vi "AddTargets.vi"(8 "error in (no error)":errorcluster, 9 "Difficulty":u8, 10 "Num Targets":i32, 11 "Level in":refnum<class "Level.lvclass">) -> (0 "error out":errorcluster, 3 "Level out":refnum<class "Level.lvclass">)   [LabVIEW 2015, in "Level.lvclass"]
uses:
  Level.lvclass
  Level.lvclass/Level.ctl
  Segment.ctl
  Point.ctl
  3D Point.ctl
  3D Object/3D Object.lvclass
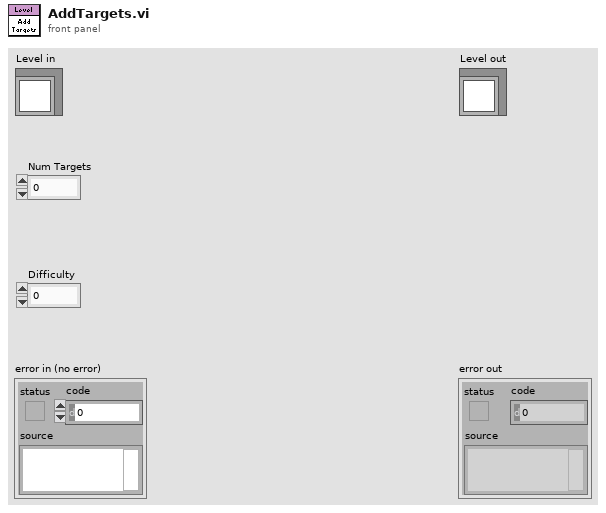
[diagram p1: front panel]
types:
  T1 = typedef "Level.lvclass/Segment.ctl" = cluster{"Point 1":T2, "Point 2":T2}
  T2 = typedef "Level.lvclass/Point.ctl" = cluster{"Z":dbl, "X":dbl}
  T3 = typedef "3D Point.ctl" = cluster{"X":sgl, "Y":sgl, "Z":sgl}
  T4 = cluster{"Collision":T1, "Position":T3, "Radius":dbl}
  T5 = enum16{"As a Decal", "With Modulation", "With Blending", "As a replacement"}
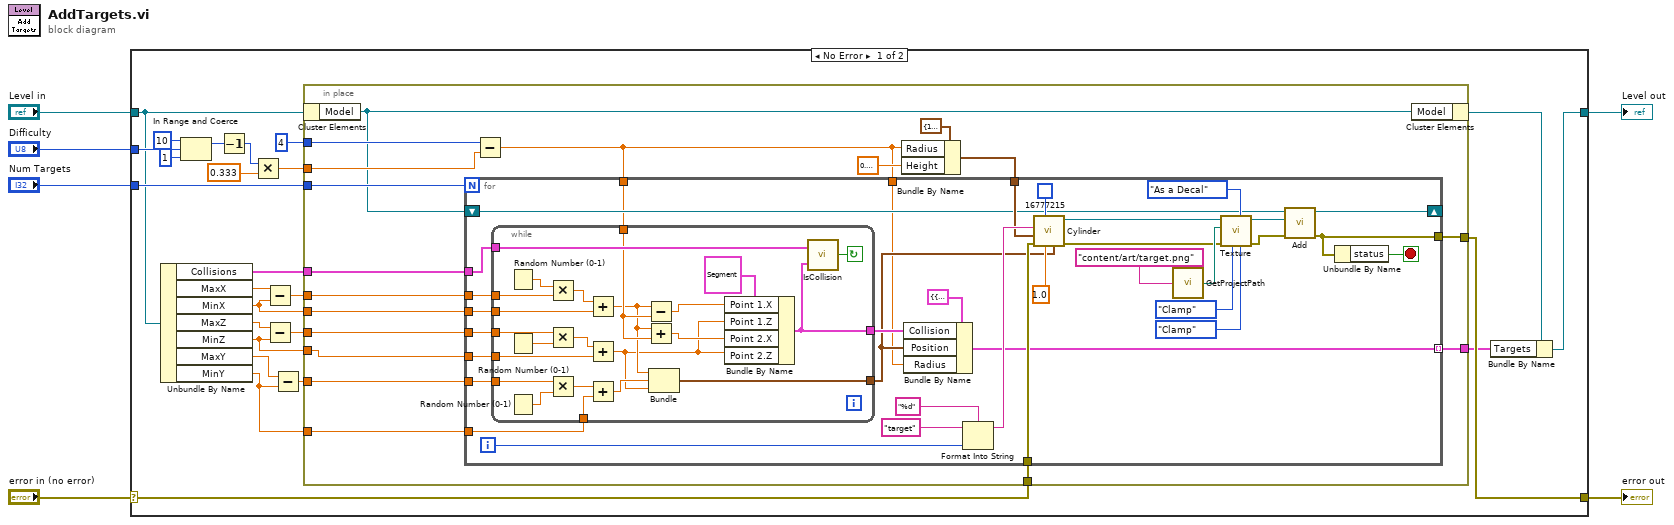
[diagram p0: block diagram]
diagram:
  n1 = case shown="No Error" "error in (no error)" {
    selector: "error in (no error)" -> [w11 w108]
    tunnel: [w12 w108] -> w5
    tunnel: [w8 w107] -> w3
    tunnel: "Level in" -> [w22 w107]
    tunnel: "Difficulty" -> [w31 _]
    tunnel: "Num Targets" -> [w28 _]
    frame No Error {
      n2 = Unbundle By Name(w22) -> ("Collisions"=w10:T1[], "MaxX"=w27:sgl, "MinX"=w24:sgl, "MaxZ"=w26:sgl, "MinZ"=w23:sgl, "MaxY"=w20:sgl, "MinY"=w18:sgl)
      n3 = In Range and Coerce(upper limit=u8 10, x=w31, lower limit=u8 1) -> (coerced(x)=w16:u8)  [unwired: 1 out]
      n4 = Decrement(x=w16) -> (x-1=w15:u8)
      n5 = Multiply(x=w15, y=0.333) -> (x*y=w13:dbl)
      n6 = Subtract(x=w27, y=w24) -> (x-y=w25:sgl)
      n7 = Subtract(x=w26, y=w23) -> (x-y=w21:sgl)
      n8 = Subtract(x=w20, y=w18) -> (x-y=w19:sgl)
      n9 = in-place {
        in-place-border: w28 -> [w49]
        in-place-border: w25 -> [w48]
        in-place-border: w21 -> [w47]
        in-place-border: w24 -> [w46]
        in-place-border: w23 -> [w45]
        in-place-border: w19 -> [w44]
        in-place-border: w18 -> [w43]
        in-place-border: 4 -> [w39]
        in-place-border: w13 -> [w38]
        in-place-border: [w37] -> w12
        in-place-border: w11 -> [w36]
        in-place-border: w10 -> [w35]
        in-place-border: [w32] -> w7
        n10 = in-place-cluster #1(w22) -> ("Model"=w34:refnum<class "3D Object.lvclass">)
        n11 = Subtract(x=w39, y=w38) -> (x-y=w33:dbl)
        n12 = Bundle By Name(cluster=cluster{"Height":sgl, "Radius":sgl} {"Height"=1.0, "Radius"=1.0} ("Size"), "Radius"=w33, "Height"=sgl 0.1) -> (w40:cluster{"Height":sgl, "Radius":sgl})
        n13 = for {
          N: w49 -> [_]
          tunnel: w48 -> [w83]
          tunnel: w47 -> [w82]
          tunnel: w46 -> [w81]
          tunnel: w45 -> [w80]
          tunnel: w44 -> [w74]
          tunnel: w43 -> [w73]
          tunnel: w40 -> [w67]
          shift-right: [w65] -> _
          shift-left: w34 -> [w64]
          tunnel: [w58] -> w37
          tunnel: w36 -> [w59]
          tunnel: w35 -> [w56]
          tunnel: w33 -> [w55]
          tunnel: w33 -> [w51]
          tunnel: [w50] -> w32 mode=indexing
          i -> [w77]
          stop <- w57 stop-if-true
          n14 = while {
            tunnel: w83 -> [w106]
            tunnel: w82 -> [w104]
            tunnel: w81 -> [w102]
            tunnel: w80 -> [w100]
            tunnel: w74 -> [w98]
            tunnel: w73 -> [w95]
            tunnel: w56 -> [w94]
            tunnel: w55 -> [w92]
            tunnel: [w90] -> w52
            tunnel: [w87] -> w53
            stop <- w93 continue-if-true
            n15 = Random Number (0-1)() -> (number: 0 to 1=w105:dbl)
            n16 = Random Number (0-1)() -> (number: 0 to 1=w103:dbl)
            n17 = Random Number (0-1)() -> (number: 0 to 1=w97:dbl)
            n18 = Multiply(x=w105, y=w106) -> (x*y=w101:dbl)
            n19 = Multiply(x=w104, y=w103) -> (x*y=w99:dbl)
            n20 = Multiply(x=w98, y=w97) -> (x*y=w96:dbl)
            n21 = Add(x=w101, y=w102) -> (x+y=w89:dbl)
            n22 = Add(x=w99, y=w100) -> (x+y=w84:dbl)
            n23 = Add(x=w96, y=w95) -> (x+y=w91:dbl)
            n24 = Subtract(x=w89, y=w92) -> (x-y=w86:dbl)
            n25 = Add(x=w89, y=w92) -> (x+y=w85:dbl)
            n26 = Bundle(w89, w91, w84) -> (w90:cluster{dbl, dbl, dbl})  [unwired: 1 in]
            n27 = Bundle By Name(cluster=T1 {"Point 1"={"Z"=-84.88052004597432, "X"=174.2806833080472}, "Point 2"={"Z"=-79.54452004597431, "X"=174.2806833080472}} ("Segment"), "Point 1.X"=w86, "Point 1.Z"=w84, "Point 2.X"=w85, "Point 2.Z"=w84) -> (w87:T1)
            n28 = call "IsCollision.vi"("Segment B"=w87, "Collisions"=w94) -> ("Collision?"=w93:bool)
          }
          n29 = Bundle By Name(cluster=T4 {"Collision"={"Point 1"={"Z"=0.0, "X"=0.0}, "Point 2"={"Z"=0.0, "X"=0.0}}, "Position"={"X"=0.0, "Y"=0.0, "Z"=0.0}, "Radius"=0.0} ("Target Data"), "Collision"=w53, "Position"=w52, "Radius"=w51) -> (w50:T4)
          n30 = Format Into String(format string="%d", initial string="target", w77) -> (resulting string=w76:string)  [unwired: 1 in, 1 out]
          n31 = call "Cylinder.vi"("Position"=w52, "Detail"=sgl 1.0, "Color Box"=u32 16777215, "error in (no error)"=w59, "Size"=w67, "Name"=w76) -> ("error out"=w60:errorcluster, "3D Object out"=w72:refnum<class "3D Object.lvclass">)  [unwired: 4 in]
          n32 = call "GetProjectPath.vi"("File"="content/art/target.png") -> ("Path"=w69:path)
          n33 = call "Texture.vi"("Vertical Wrap Mode"=enum16{"Clamp", "Repeat"}."Clamp", "Apply Mode"=T5."As a Decal", "Horizontal Wrap Mode"=enum16{"Clamp", "Repeat"}."Clamp", "error in (no error)"=w60, "path to image"=w69, "Object in"=w72) -> ("error out"=w61:errorcluster, "Object out"=w71:refnum<class "3D Object.lvclass">)  [unwired: 4 in]
          n34 = call "Add.vi"("error in (no error)"=w61, "Child in"=w71, "Parent in"=w64) -> ("error out"=w58:errorcluster, "Parent out"=w65:refnum<class "3D Object.lvclass">)  [unwired: 6 in, 1 out]
          n35 = Unbundle By Name(w58) -> ("status"=w57:bool)
        }
        n36 = in-place-cluster #1("Model"=w34) -> (w9:refnum<class "Level.lvclass">)
      }
      n37 = Bundle By Name(cluster=w9, "Targets"=w7) -> (w8:refnum<class "Level.lvclass">)
    }
    frame Error {
    }
  }
  "error out" <- w5
  "Level out" <- w3
